vi "3D_plot.vi"() -> ()   [LabVIEW 2013]
uses:
  <vilib>/Native 3D Graph/xcontrol/3DPC_SurfacePlot.xctl
panel:
  in  "Y-step":i32
  in  "Subtract?":bool
  in  "Filename":path=path "test.lvm"
  out "?":refnum<class "Base Datatype.lvclass">[](xcontrol)
  in  "Subtract Value":dbl
  in  "X-step":i32
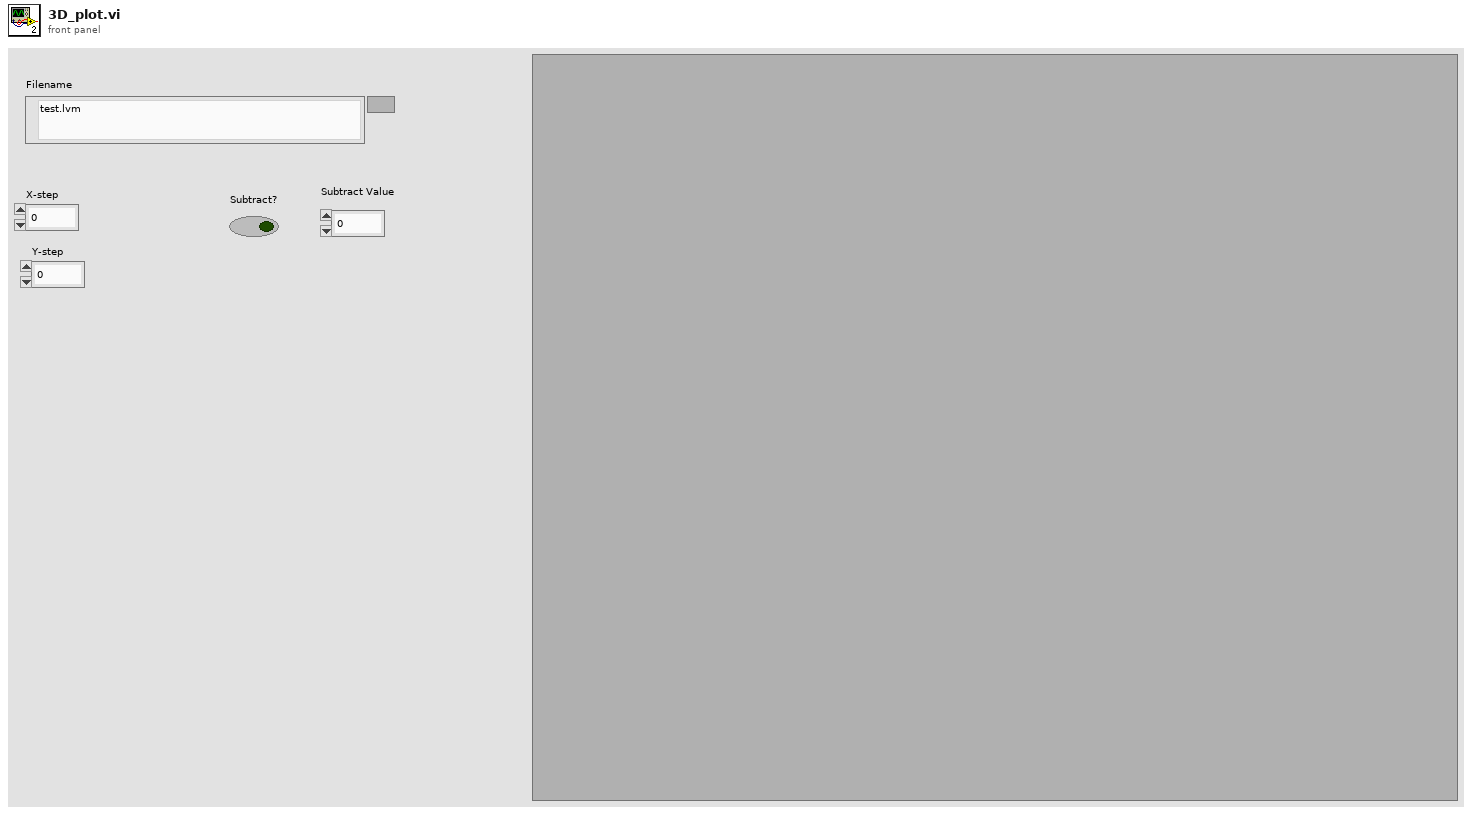
[diagram p1: front panel]
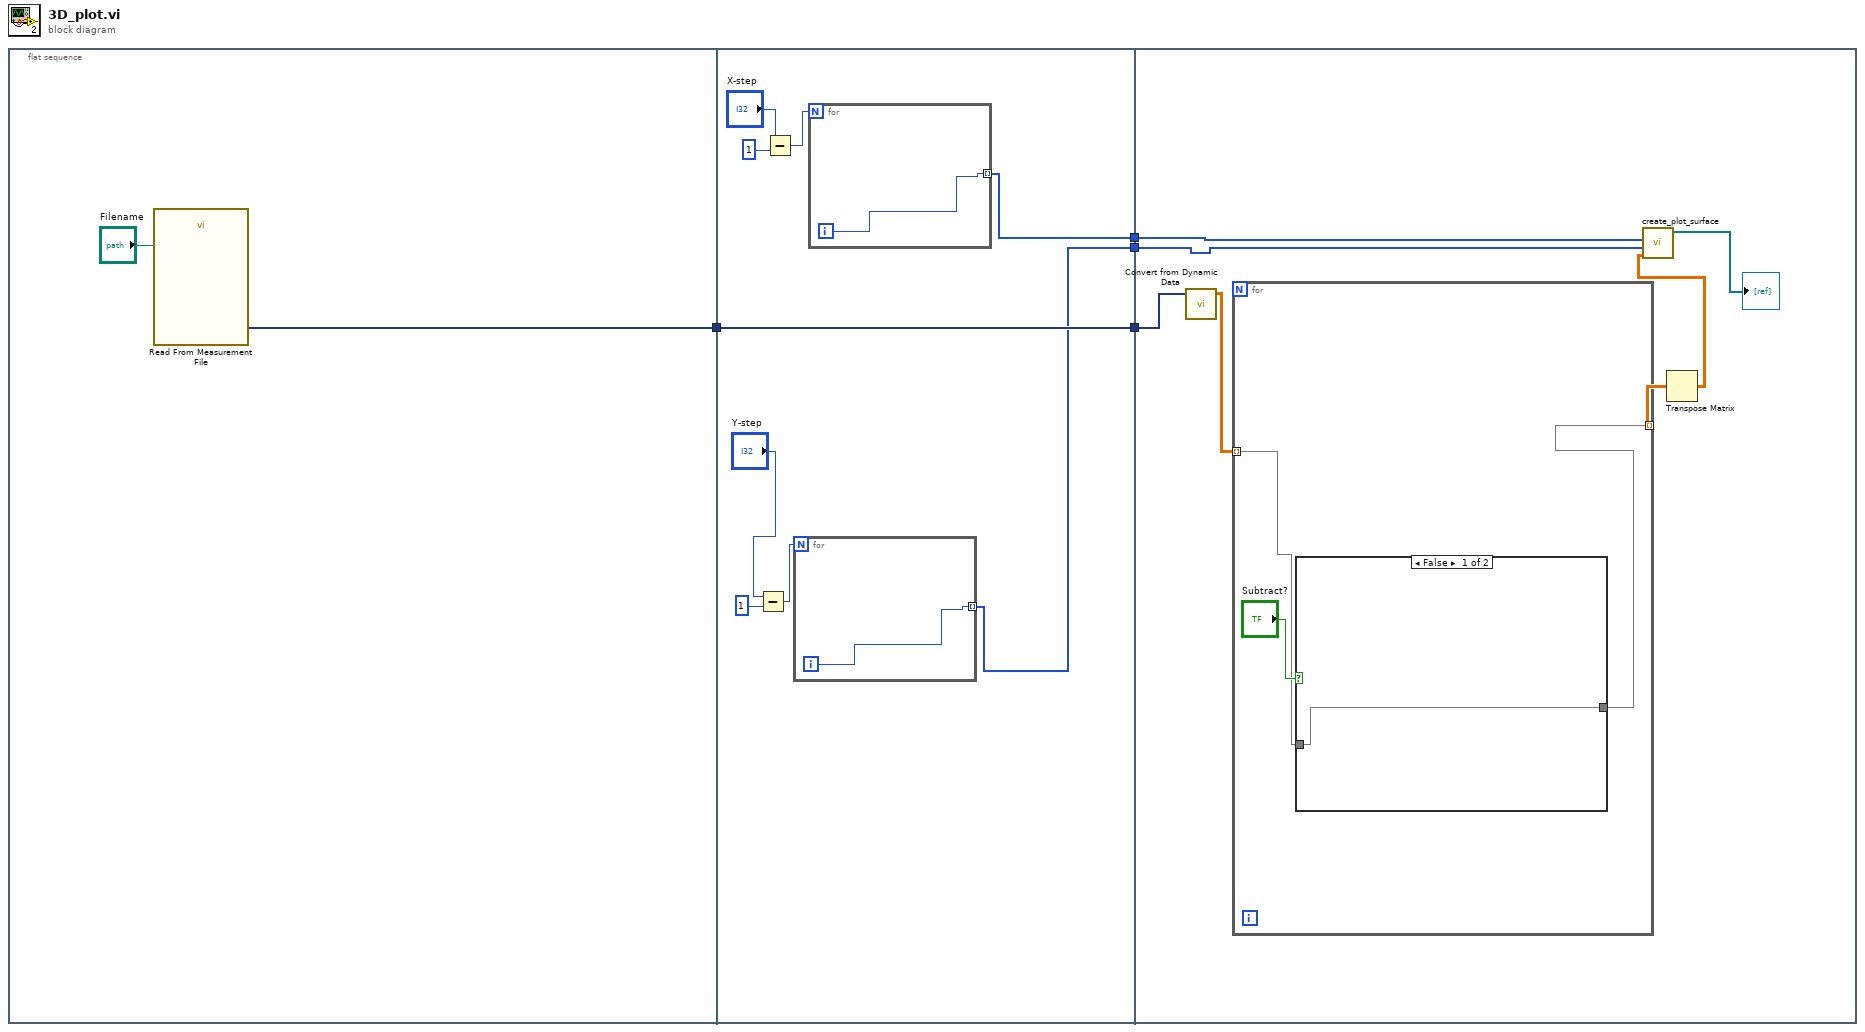
[diagram p0: block diagram]
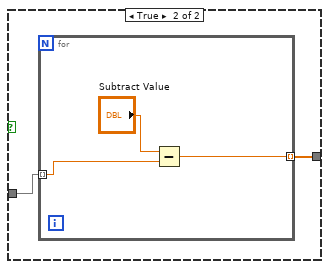
[diagram p2: hidden frame]
diagram:
  n1 = flat-sequence {
    tunnel: [w6] -> w2
    tunnel: [w15] -> w4
    tunnel: [w14] -> w3
    tunnel: w2 -> [w14]
    tunnel: [w13] -> w1
    tunnel: w4 -> [w24]
    tunnel: w3 -> [w23]
    tunnel: w1 -> [w18]
    frame #0 {
      n2 = call "Read From Measurement File"("Filename"="Filename") -> ("Signals"=w6:dynamicdata)  [unwired: 5 in, 5 out]
    }
    frame #1 {
      n3 = Subtract(x="Y-step", y=1) -> (x-y=w7:i32)
      n4 = Subtract(x="X-step", y=1) -> (x-y=w10:i32)
      n5 = for {
        N: w7 -> [_]
        tunnel: [w16] -> w13 mode=indexing
        i -> [w16]
      }
      n6 = for {
        N: w10 -> [_]
        tunnel: [w17] -> w15 mode=indexing
        i -> [w17]
      }
    }
    frame #2 {
      n7 = call "Convert from Dynamic Data"("Dynamic Data Type"=w23) -> ("Array"=w22:dbl[][])  [unwired: 3 in]
      n8 = for {
        tunnel: w22 -> [w26] mode=indexing
        tunnel: [w25] -> w20 mode=indexing
        n9 = case shown="False" "Subtract?" {
          tunnel: w26 -> [w28 w30]
          tunnel: [w28 w29] -> w25
          frame False {
          }
          frame True {
            n10 = for {
              tunnel: w30 -> [w33] mode=indexing
              tunnel: [w32] -> w29 mode=indexing
              n11 = Subtract(x="Subtract Value", y=w33) -> (x-y=w32:dbl)
            }
          }
        }
      }
      n12 = Transpose Matrix(1:w20) -> (0:w19:dbl[][])
      n13 = call <vilib>:"create_plot_surface.vi"("z matrix"=w19, "y vector"=w18, "x vector"=w24) -> ("plots out"=→"?":refnum<class "Base Datatype.lvclass">[])  [unwired: 2 in, 6 out]
    }
  }
